vi "img.saveIndividual.EL.vi"(5 "vars":T1={"save"={"base_folder"={"Folder"=path "", "tif"=FALSE, "jpg"=FALSE}, "module"="", "#"=20, "sub#"=0, "save.op"=enum."Full", "same?"=FALSE, "Shift"=enum."Single", "jpg?"=FALSE, "flip"={"x"=FALSE, "y"=FALSE}}, "acq"={"# Acq"=100, "rotate"=FALSE}, "calib.manual"={"BG"={"Image"=[], "enabled?"=FALSE}, "FF"={"Image"=[], "enabled?"=FALSE}}}, 6 "loop":i32, 7 "path":path, 8 "error in":errorcluster, 10 "EL":u16[][](array[numeric])) -> (0 "error out":errorcluster)   [LabVIEW 2020]
uses:
  _controls/data.vars.ctl
  _controls/flip.ctl
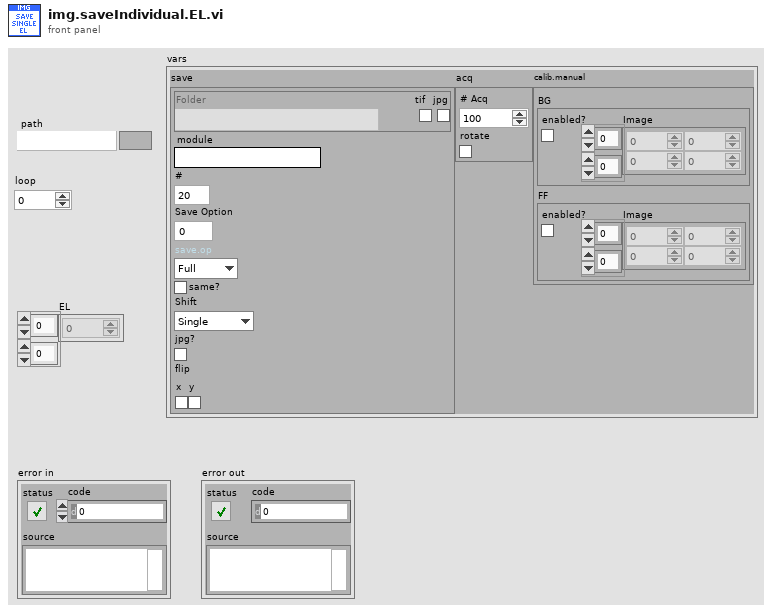
[diagram p1: front panel]
types:
  T1 = typedef "data.vars.ctl" = cluster{"save":cluster{"base_folder":cluster{"Folder":path, "tif":bool, "jpg":bool}, "module":string, "#":u32, "sub#":u8, "save.op":enum16{"Full", "Light"}, "same?":bool, "Shift":enum16{"Single", "Leapfrog"}, "jpg?":bool, "flip":T2}, "acq":cluster{"# Acq":u16, "rotate":bool}, "calib.manual":cluster{"BG":cluster{"Image":u16[][], "enabled?":bool}, "FF":cluster{"Image":u16[][], "enabled?":bool}}}
  T2 = typedef "flip.ctl" = cluster{"x":bool, "y":bool}
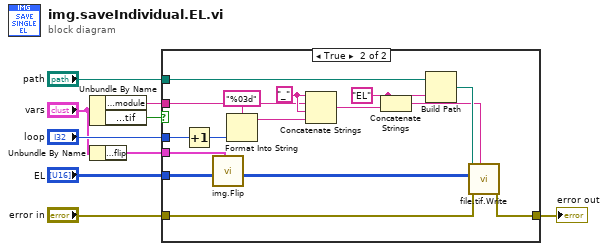
[diagram p0: block diagram]
diagram:
  n1 = Unbundle By Name("vars") -> ("save.module"=w4:string, "save.base_folder.tif"=w3:bool)
  n2 = Unbundle By Name("vars") -> ("save.flip"=w1:T2)
  n3 = case shown="True" w3 {
    tunnel: "EL" -> [_ w14]
    tunnel: "error in" -> [w10 w26]
    tunnel: "path" -> [_ w19]
    tunnel: [w10 w11] -> w6
    tunnel: "loop" -> [_ w18]
    tunnel: w4 -> [_ w17]
    tunnel: w1 -> [_ w12]
    frame False {
    }
    frame True {
      w25 = "EL" ("String")
      w20 = "_" ("string")
      n4 = Increment(x=w18) -> (x+1=w24:i32)
      n5 = call "img.Flip.vi"("flip"=w12, "image in"=w14) -> ("image out"=w13:u16[][])  [unwired: 9 in]
      n6 = Format Into String(format string="%03d", w24) -> (resulting string=w22:string)  [unwired: 2 in, 1 out]
      n7 = Concatenate Strings(w20, w17, w20, w22) -> (w21:string)
      n8 = Concatenate Strings(w25, w21) -> (w15:string)
      n9 = Build Path(base path=w19, name or relative path=w25) -> (appended path=w16:path)
      n10 = call "file.tif.Write.vi"("name"=w15, "error in"=w26, "u16 pixmap"=w13, "path"=w16) -> ("error out"=w11:errorcluster)  [unwired: 7 in]
    }
  }
  "error out" <- w6
